vi "Red Pitaya Manager.vi"() -> ()   [LabVIEW 2021]
uses:
  NHMFL_Core/Libraries/Red Pitaya/Red Pitaya Digitizer/Red Pitaya Digitizer.lvclass
  NHMFL_Core/Libraries/Instruments/Pulse Driver/Pusle Driver Configuration.ctl
panel:
  out "Armed":bool
  out "Tranfer speed":dbl format="%#_6pbytes/s"
  out "Total time":dbl format="%#_gs"
  in  "Configuration":T1={"Post-trigger delay"=0.01, "Post-trigger duration"=0.1, "Rate"=125000000.0, "Ranges"=[1.0], "Re-name channels"=["V1", "V2"], "Active channels"="0:1", "External clock"=FALSE} {"Rate" format="%#_8pHz"; "Post-trigger duration" format="%#_6ps"; "Post-trigger delay" format="%#_6ps"; "Ranges" format="%#_6pV"}
  in  "Speed test":bool
  in  "FPGA Logic":T2(ring)
  in  "Exir":bool
  in  "Red Pitaya addresses":i32(listbox)
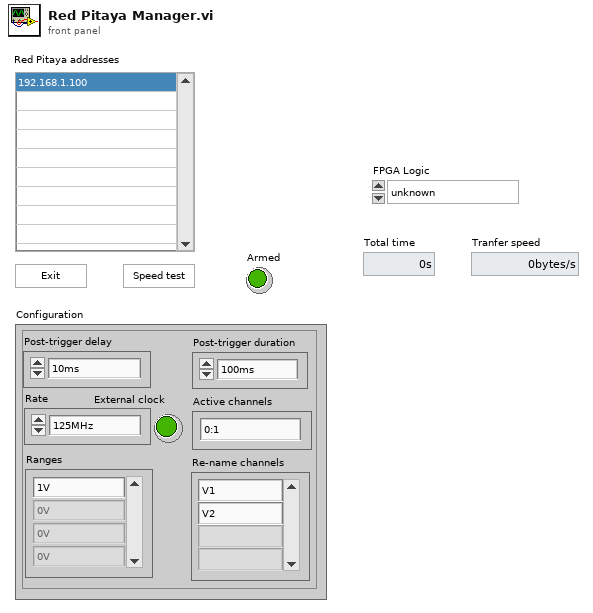
[diagram p1: front panel]
types:
  T1 = typedef "Pusle Driver Configuration.ctl" = cluster{"Post-trigger delay":dbl, "Post-trigger duration":dbl, "Rate":dbl, "Ranges":dbl[], "Re-name channels":string[], "Active channels":string, "External clock":bool}
  T2 = enum16{"unknown", "lockin_sweep", "current_voltage", "syncronous_lockin", "single_channel_lockin"}
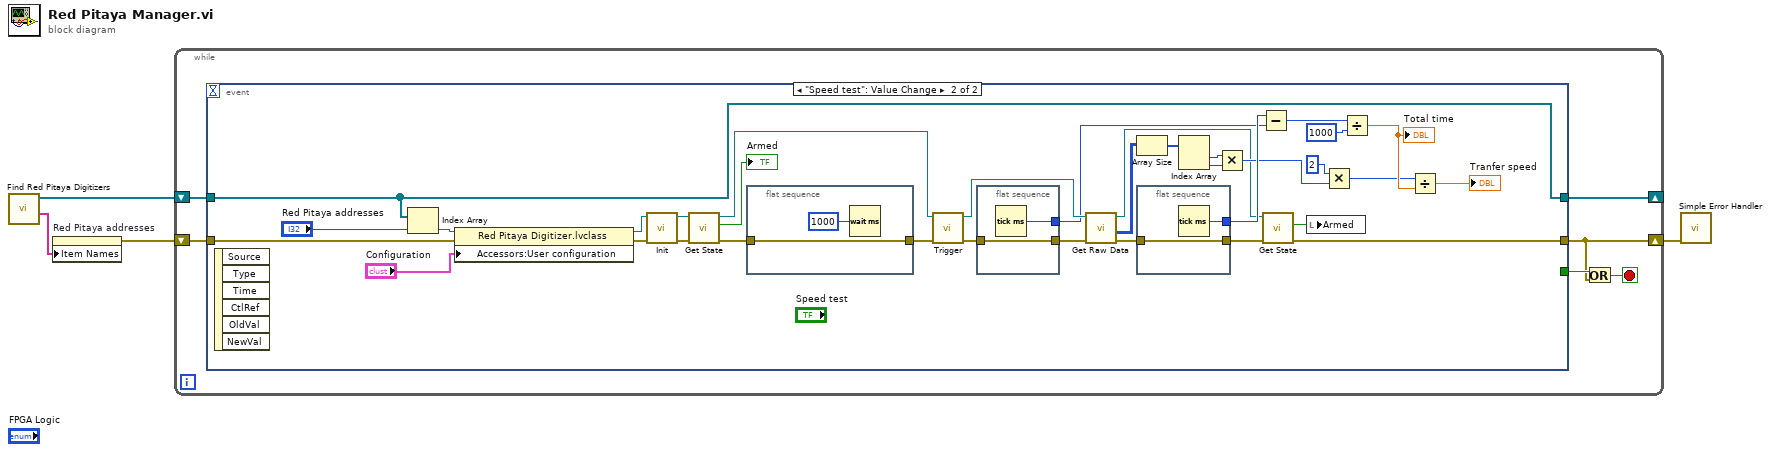
[diagram p0: block diagram]
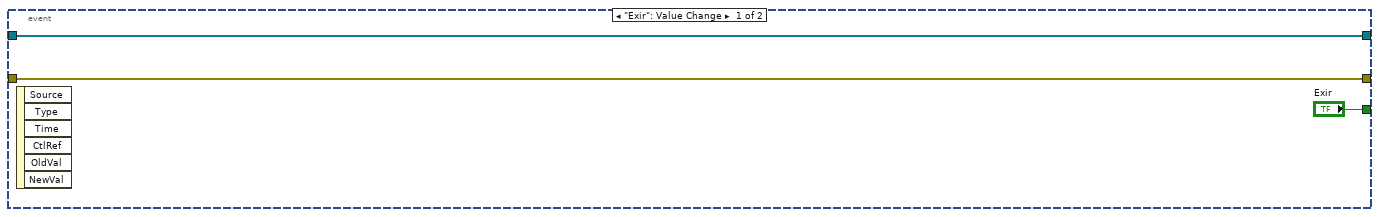
[diagram p2: hidden frame]
diagram:
  n1 = call "Find Red Pitaya Digitizers.vi"() -> ("Addresses"=w3:string[], "Digitizers out"=w2:refnum<class "Red Pitaya Digitizer.lvclass">[])  [unwired: 8 in, 2 out]
  n2 = property on="Red Pitaya addresses" class="LstBox (strict)"("Item Names"=w3) -> (error out=w4:errorcluster)  [unwired: 2 in, 1 out]
  n3 = while {
    shift-right: [w7] -> _
    shift-left: w2 -> [w8]
    shift-right: [w5] -> w1
    shift-left: w4 -> [w9]
    stop <- w6 stop-if-true
    n4 = event shown="[1] \"Speed test\": Value Change" {
      selector: _ -> [_ _]
      dyn-events: _ -> [_ _]
      timeout: _ -> [_ _]
      tunnel: ["Exir" _] -> w10
      tunnel: w9 -> [w11 w42]
      tunnel: w8 -> [w12 w45]
      tunnel: [w12 w45] -> w7
      tunnel: [w11 w15] -> w5
      event "Exir": Value Change {
        n5 = event-data() -> ()  [unwired: 1 in, 6 out]
      }
      event "Speed test": Value Change {
        n6 = event-data() -> ()  [unwired: 1 in, 6 out]
        n7 = Index Array(array=w45, index="Red Pitaya addresses") -> (element=w46:refnum<class "Red Pitaya Digitizer.lvclass">)
        n8 = property class="Red Pitaya Digitizer.lvclass"(reference=w46, error in=w42, "Accessors:User configuration"="Configuration") -> (reference out=w44:refnum<class "Red Pitaya Digitizer.lvclass">, error out=w41:errorcluster)
        n9 = call-dynamic "Init.vi"("error in (no error)"=w41, "Instrument Driver in"=w44) -> ("error out"=w21:errorcluster, "Instrument Driver out"=w22:refnum<class "Red Pitaya Digitizer.lvclass">)  [unwired: 6 in, 2 out]
        n10 = call-dynamic "Get State.vi"("error in (no error)"=w21, "Red Pitaya Digitizer in"=w22) -> ("error out"=w20:errorcluster, "Armed"=→"Armed":bool, "Red Pitaya Digitizer out"=w19:refnum<class "Red Pitaya Digitizer.lvclass">)  [unwired: 4 in, 3 out]
        n11 = flat-sequence {
          tunnel: w20 -> [w49]
          tunnel: [w49] -> w23
          frame #0 {
            n12 = Wait (ms)(milliseconds to wait=u32 1000) -> ()  [unwired: 1 out]
          }
        }
        n13 = call-dynamic "Trigger.vi"("error in (no error)"=w23, "Red Pitaya Digitizer in"=w19) -> ("error out"=w39:errorcluster, "Red Pitaya Digitizer out"=w40:refnum<class "Red Pitaya Digitizer.lvclass">)  [unwired: 8 in]
        n14 = flat-sequence {
          tunnel: w39 -> [w52]
          tunnel: [w52] -> w37
          tunnel: [w53] -> w35
          frame #0 {
            n15 = Tick Count (ms)() -> (millisecond timer value=w53:u32)
          }
        }
        n16 = call-dynamic "Get Raw Data.vi"("error in (no error)"=w37, "Red Pitaya Digitizer in"=w40) -> ("error out"=w38:errorcluster, "appended array"=w32:i16[][], "Red Pitaya Digitizer out"=w17:refnum<class "Red Pitaya Digitizer.lvclass">)  [unwired: 7 in]
        n17 = Array Size(array=w32) -> (size(s)=w31:i32[])
        n18 = flat-sequence {
          tunnel: w38 -> [w51]
          tunnel: [w51] -> w16
          tunnel: [w50] -> w36
          frame #0 {
            n19 = Tick Count (ms)() -> (millisecond timer value=w50:u32)
          }
        }
        n20 = Index Array(array=w31) -> (element #1=w30:i32, element #2=w29:i32)  [unwired: 2 in]
        n21 = Multiply(x=w30, y=w29) -> (x*y=w25:i32)
        n22 = Subtract(x=w36, y=w35) -> (x-y=w34:u32)
        n23 = call-dynamic "Get State.vi"("error in (no error)"=w16, "Red Pitaya Digitizer in"=w17) -> ("error out"=w15:errorcluster, "Armed"=w14:bool)  [unwired: 4 in, 4 out]
        n24 = local write "Armed"(w14) -> ()
        n25 = Multiply(x=2, y=w25) -> (x*y=w26:i32)
        n26 = Divide(x=w34, y=u32 1000) -> (x/y=w27:dbl)
        "Total time" <- w27
        n27 = Divide(x=w26, y=w27) -> (x/y=→"Tranfer speed":dbl)
      }
    }
    n28 = Or(x=w10, y=w5) -> (x .or. y?=w6:bool)
  }
  n29 = call <vilib>:"Simple Error Handler.vi"("error in (no error)"=w1) -> ()  [unwired: 4 in, 5 out]
